vi "GenXML.vi"(9 "dateTo":string, 10 "dateFrom":string, 11 "file name":path) -> (1 "Application Directory":path, 2 "connection information":path, 3 "error out":errorcluster)   [LabVIEW 2014]
doc: "Used to extract XML file from Transactions Table between dates selected (from-to)"
uses:
  <vilib>/addons/database/Recordset.llb/Rec Save Format.ctl
  <vilib>/addons/database/Connection.llb/DB Tools Open Connec (Path).vi
  <vilib>/addons/database/Connection.llb/Conn Execute.vi
  <vilib>/addons/database/Recordset.llb/Rec Save Recordset To File (R).vi
  <vilib>/addons/database/NI_Database_API.lvlib
panel:
  # "used to generate XML File for Transactions"
  # "Inputs"
  # "Outputs"
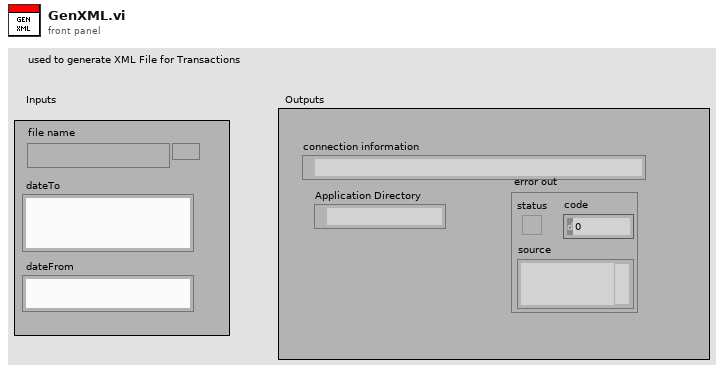
[diagram p1: front panel]
types:
  T1 = typedef "NI_Database_API.lvlib/Rec Save Format.ctl" = enum16{"ADTG", "XML"}
  T2 = typedef "NI_Database_API.lvlib/Conn ObjectReference.ctl" = refnum<k1>
  T3 = typedef "NI_Database_API.lvlib/Rec ObjectReference.ctl" = refnum<k1>
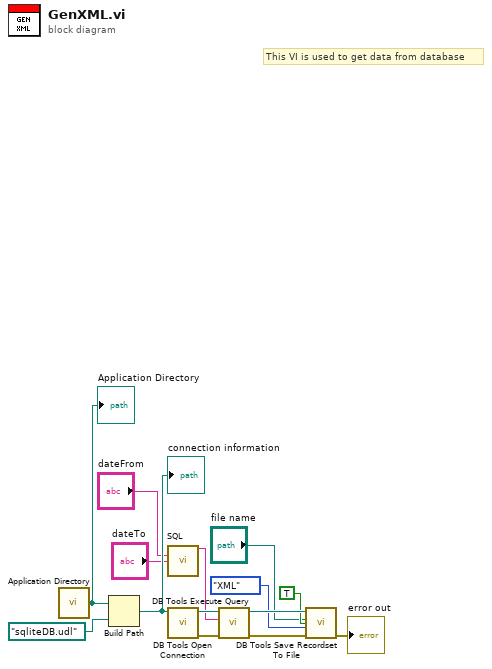
[diagram p0: block diagram]
diagram:
  # "This VI is used to get data from database"
  n1 = call <vilib>:"Application Directory.vi"() -> ("Application Directory"=w14:path)
  "Application Directory" <- w14
  n2 = Build Path(base path=w14, name or relative path=path "sqliteDB.udl" ("connection information")) -> (appended path=w13:path)
  "connection information" <- w13
  n3 = call "SQL"("dateFrom"="dateFrom", "dateTo"="dateTo") -> ("Result"=w5:string)  [unwired: 12 in, 1 out]
  n4 = call-poly <vilib>:"DB Tools Open Connection.vi"("connection information"=w13) -> ("error out"=w6:errorcluster, "connection reference"=w7:T2)  [unwired: 7 in]
  n5 = call-poly <vilib>:"DB Tools Execute Query.vi"("error in (no error)"=w6, "SQL query"=w5, "connection reference"=w7) -> ("error out"=w9:errorcluster, "recordset reference"=w11:T3)  [unwired: 5 in]
  n6 = call-poly <vilib>:"DB Tools Save Recordset To File.vi"("overwrite? (F)"=TRUE, "error in (no error)"=w9, "save format (XML)"=Rec_Save_Format."XML", "file name"="file name", "recordset reference"=w11) -> ("error out"=→"error out":errorcluster)  [unwired: 3 in, 1 out]
